vi "TestingTypeNames.vi"() -> ()   [LabVIEW 2017]
panel:
  out "ToString":string
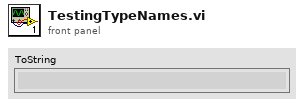
[diagram p1: front panel]
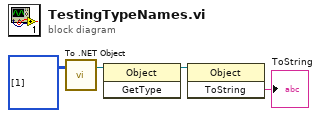
[diagram p0: block diagram]
diagram:
  n1 = call <vilib>:"To .NET Object.vi"("anything"=i32[][][] [[[1]]]) -> (".NET object"=w3:refnum<k24>)  [unwired: 1 in, 1 out]
  n2 = invoke class="Object" method="GetType"(reference=w3) -> (reference out=w2:refnum<k24>)  [unwired: 2 in, 2 out]
  n3 = invoke class="Object" method="ToString"(reference=w2) -> ("ToString"=→"ToString":string)  [unwired: 2 in, 2 out]
